vi "GetControlClass.vi"(5 "name":string, 6 "error in":errorcluster, 9 "PythonConverter_GUI in":refnum<class "PythonConverter_GUI.lvclass">) -> (0 "error out":errorcluster, 3 "PythonConverter_GUI out":refnum<class "PythonConverter_GUI.lvclass">, 4 "class":string)   [LabVIEW 2014, in "PythonConverter_GUI.lvclass"]
uses:
  PythonConverter_GUI.lvclass
  PythonConverter_GUI.lvclass/PythonConverter_GUI.ctl
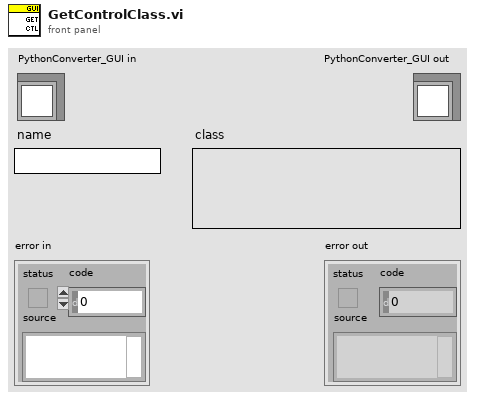
[diagram p1: front panel]
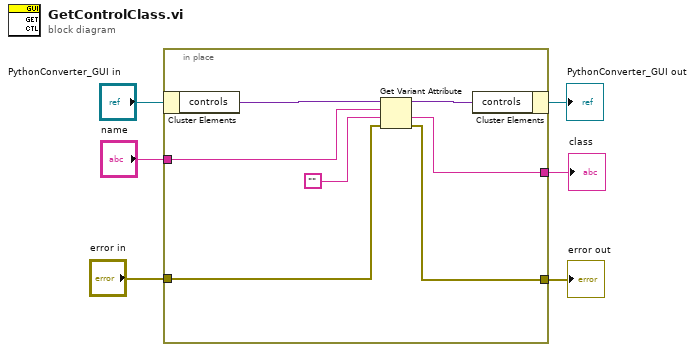
[diagram p0: block diagram]
diagram:
  n1 = in-place {
    in-place-border: "error in" -> [w11]
    in-place-border: [w10] -> w4
    in-place-border: "name" -> [w9]
    in-place-border: [w8] -> w1
    n2 = in-place-cluster #1("PythonConverter_GUI in") -> ("controls"=w13:variant)
    n3 = Get Variant Attribute(Variant=w13, name=w9, default value (empty Variant)="", error in=w11) -> (duplicate Variant=w12:variant, value=w8:string, error out=w10:errorcluster)  [unwired: 1 out]
    n4 = in-place-cluster #1("controls"=w12) -> (→"PythonConverter_GUI out":refnum<class "PythonConverter_GUI.lvclass">)
  }
  "error out" <- w4
  "class" <- w1
